vi "Create File.vi"(9 "Column Titles":string[](array[string]), 11 "File Name":string) -> (2 "File Reference Out":refnum<file>)   [LabVIEW 2016]
uses:
  Global Variables/Folder Names.vi
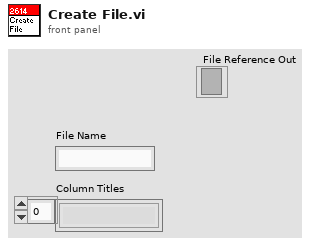
[diagram p1: front panel]
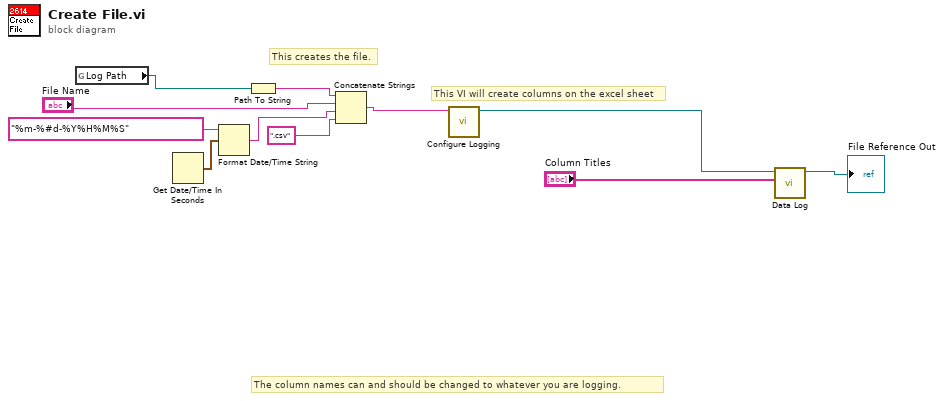
[diagram p0: block diagram]
diagram:
  # "The column names can and should be changed to whatever you are logging."
  # "This VI will create columns on the excel sheet"
  # "This creates the file."
  n1 = global read "Folder Names.vi" "Log Path"() -> (w10:path)
  n2 = Get Date/Time In Seconds() -> (seconds since 1Jan1904=w6:timestamp)
  n3 = Format Date/Time String(time format string (%c)="%m-%#d-%Y%H%M%S", seconds (now)=w6) -> (date/time string=w4:string)  [unwired: 1 in]
  n4 = Path To String(path=w10) -> (string=w9:string)
  n5 = Concatenate Strings(w9, "File Name", w4, ".csv" ("string")) -> (w11:string)
  n6 = call "Configure Logging.vi"("File Path/File Name"=w11) -> ("refnum out"=w8:refnum<file>)  [unwired: 10 in]
  n7 = call "Data Log.vi"("Data In"="Column Titles", "File Reference In"=w8) -> ("File Reference Out"=→"File Reference Out":refnum<file>)  [unwired: 9 in]
